vi "打印报表.vi"(1 "成员信息":string, 2 "?":bool) -> (0 "?":cluster{"初始x轴值":i32, "△X":i32, i64[][]}(graph))   [LabVIEW 2016]
uses:
  <vilib>/Utility/file.llb/Read Delimited Spreadsheet (I64).vi
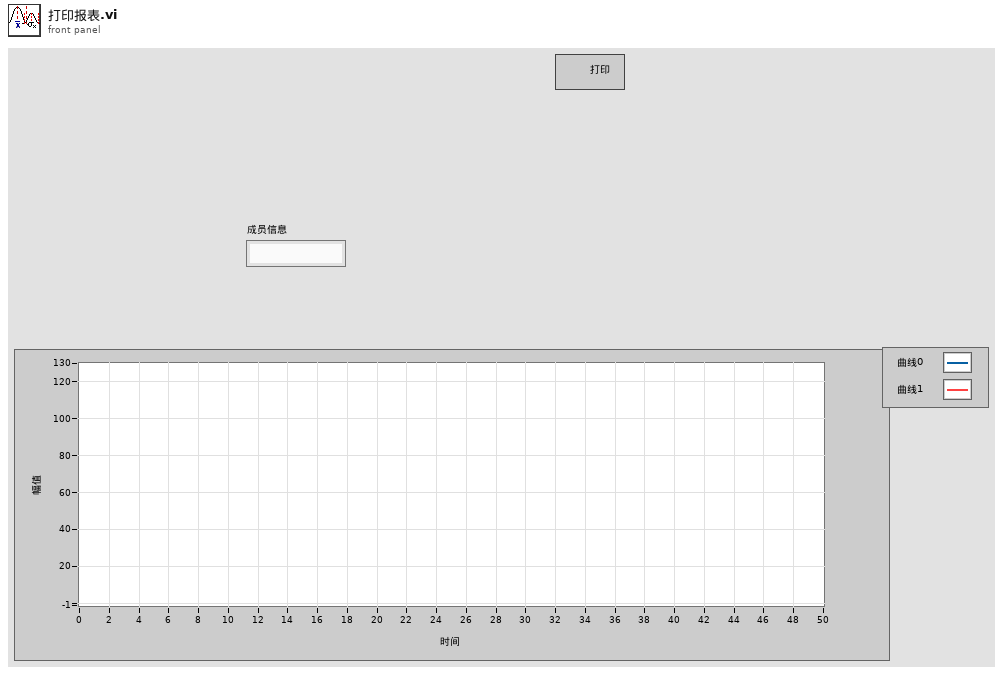
[diagram p1: front panel]
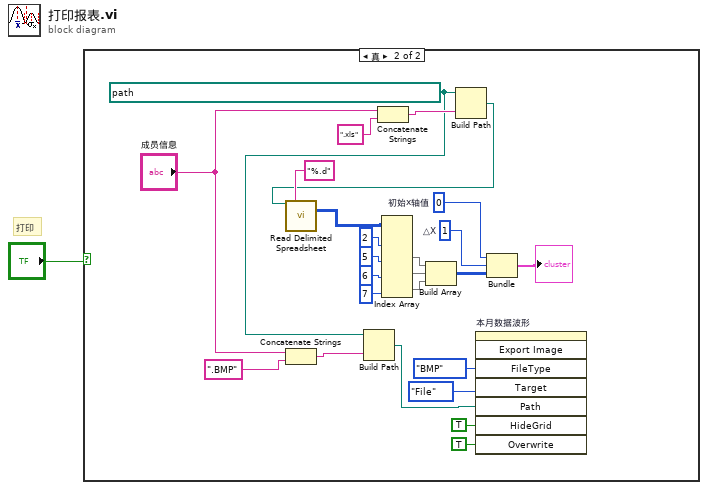
[diagram p0: block diagram]
diagram:
  # "打印"
  n1 = case shown="真" "?" {
    frame False {
    }
    frame True {
      w12 = 1  # △X
      w13 = 0  # 初始x轴值
      w5 = path "C:/Users/Administrator/Desktop/课程设计/本月数据记录" ("基路径")
      n2 = Concatenate Strings("成员信息", ".BMP" ("字符串")) -> (w6:string)
      n3 = Build Path(base path=w5, name or relative path=w6) -> (appended path=w4:path)
      n4 = Concatenate Strings("成员信息", ".xls" ("字符串")) -> (w25:string)
      n5 = Build Path(base path=w5, name or relative path=w25) -> (appended path=w11:path)
      n6 = call-poly <vilib>:"Read Delimited Spreadsheet.vi"("file path (dialog if empty)"=w11, "format (%d)"="%.d" ("format (%.3f)")) -> ("all rows"=w23:i64[][])  [unwired: 8 in, 5 out]
      n7 = Index Array(array=w23, index (col) #1=2 ("禁用的索引 (列)"), index (col) #2=5 ("索引 (列)"), index (col) #3=6 ("索引 (列)"), index (col) #4=7 ("索引 (列)")) -> (element #2=w18:i64[], element #3=w17:i64[], element #4=w16:i64[])  [unwired: 4 in, 1 out]
      n8 = Build Array(w18, w17, w16) -> (w15:i64[][])
      n9 = invoke on="本月数据波形" class="WFGraph (严格)" method="Export Image"("FileType"=enum32{"BMP", "EPS", "EMF", "PICT"}."BMP" ("文件类型"), "Target"=enum32{"File", "Clipboard"}."File" ("目标"), "Path"=w4, "HideGrid"=TRUE ("隐藏网格"), "Overwrite"=TRUE ("始终覆盖")) -> ()  [unwired: 3 in, 8 out]
      n10 = Bundle("初始x轴值"=w13, "△X"=w12, w15) -> (→"?":cluster{"初始x轴值":i32, "△X":i32, i64[][]})  [unwired: 1 in]
    }
  }
